vi "NIlib_to_b64.vi"(1 "string in":string) -> (0 "base64 out":string)   [LabVIEW 2020]
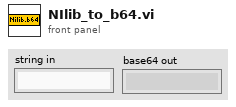
[diagram p1: front panel]
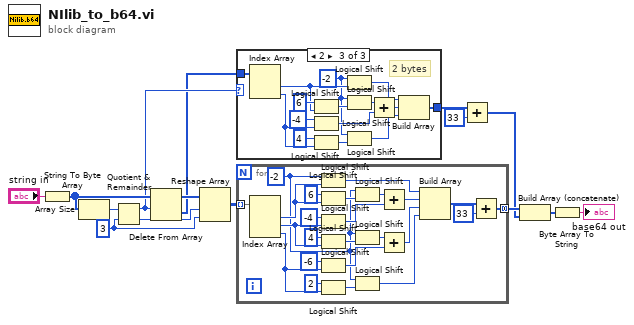
[diagram p0: block diagram]
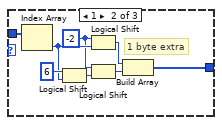
[diagram p3: hidden frame]
diagram:
  w14 = 3 ("y")
  n1 = String To Byte Array(string="string in") -> (unsigned byte array=w11:u8[])
  n2 = Array Size(array=w11) -> (size(s)=w12:i32)
  n3 = Quotient & Remainder(x=w12, y=w14) -> (x-y*floor(x/y)=w9:i32, floor(x/y)=w13:i32)
  n4 = Delete From Array(array=w11, length=w9) -> (deleted portion=w6:u8[], array with subset deleted=w15:u8[])  [unwired: 1 in]
  n5 = Reshape Array(w15, w13, w14) -> (w10:u8[][])
  n6 = case shown="2" w9 {
    tunnel: w6 -> [_ w23 w38]
    tunnel: [_ w22 w37] -> w5
    frame 0, Default {
    }
    frame 1 {
      w18 = i16 -2 ("y")
      # "1 byte extra"
      n7 = Index Array(array=w23) -> (element=w19:u8)  [unwired: 1 in]
      n8 = Logical Shift(y=i16 6, x=w19) -> (x << y=w21:u8)
      n9 = Logical Shift(y=w18, x=w19) -> (x << y=w17:u8)
      n10 = Logical Shift(y=w18, x=w21) -> (x << y=w16:u8)
      n11 = Build Array(w17, w16) -> (w22:u8[])
    }
    frame 2 {
      w25 = i16 -2 ("y")
      # "2 bytes"
      n12 = Index Array(array=w38) -> (element #1=w34:u8, element #2=w27:u8)  [unwired: 2 in]
      n13 = Logical Shift(y=i16 6, x=w34) -> (x << y=w36:u8)
      n14 = Logical Shift(y=i16 -4, x=w27) -> (x << y=w30:u8)
      n15 = Logical Shift(y=i16 4, x=w27) -> (x << y=w26:u8)
      n16 = Logical Shift(y=w25, x=w34) -> (x << y=w33:u8)
      n17 = Logical Shift(y=w25, x=w36) -> (x << y=w31:u8)
      n18 = Logical Shift(y=w25, x=w26) -> (x << y=w24:u8)
      n19 = Add(x=w31, y=w30) -> (x+y=w29:u8)
      n20 = Build Array(w33, w29, w24) -> (w37:u8[])
    }
  }
  n21 = for {
    tunnel: w10 -> [w62] mode=indexing
    tunnel: [w39] -> w8 mode=concatenating
    w43 = i16 -2 ("y")
    n22 = Index Array(array=w62) -> (element #1=w60:u8, element #2=w52:u8, element #3=w45:u8)  [unwired: 3 in]
    n23 = Logical Shift(y=w43, x=w60) -> (x << y=w55:u8)
    n24 = Logical Shift(y=i16 6, x=w60) -> (x << y=w57:u8)
    n25 = Logical Shift(y=i16 -4, x=w52) -> (x << y=w58:u8)
    n26 = Logical Shift(y=i16 4, x=w52) -> (x << y=w51:u8)
    n27 = Logical Shift(y=i16 -6, x=w45) -> (x << y=w48:u8)
    n28 = Logical Shift(y=i16 2, x=w45) -> (x << y=w44:u8)
    n29 = Logical Shift(y=w43, x=w57) -> (x << y=w56:u8)
    n30 = Logical Shift(y=w43, x=w51) -> (x << y=w49:u8)
    n31 = Logical Shift(y=w43, x=w44) -> (x << y=w42:u8)
    n32 = Add(x=w56, y=w58) -> (x+y=w54:u8)
    n33 = Add(x=w49, y=w48) -> (x+y=w47:u8)
    n34 = Build Array(w55, w54, w47, w42) -> (w41:u8[])
    n35 = Add(x=w41, y=u8 33 ("x")) -> (x+y=w39:u8[])
  }
  n36 = Add(x=w5, y=u8 33 ("x")) -> (x+y=w3:u8[])
  n37 = Build Array (concatenate)(w8, w3) -> (w7:u8[])
  n38 = Byte Array To String(unsigned byte array=w7) -> (string=→"base64 out":string)
